vi "Get Settings.vi"(6 "wait for reply (T)":bool=TRUE, 8 "error in":errorcluster) -> (0 "error out":errorcluster, 1 "timed out?":bool, 3 "Main":T4={"Heat"={"KPтерм"=8.0, "TNтерм"=12.0, "KPниз"=4.0, "TNниз"=8.0, "COM ADC"="", "COM Termex"="", "KPдд"=4.0, "TNдд"=8.0, "Multiper"=1.0}, "Расчёты"={"Vm0"=8.0, "aa"=8.0, "bb"=8.0, "K0"=8.0, "A"=8.0, "B"=8.0}, "Видеосистема"=FALSE, "Anton Paar"={"IP adress"="192.168.0.110"}, "MIDA COM"="COM11"} {"Расчёты"."B" min=0.0 max=150.0 format="%.8f"; "Расчёты"."A" min=0.0 max=150.0 format="%.8f"; "Расчёты"."K0" min=0.0 max=150.0 format="%.2f"; "Расчёты"."bb" min=0.0 max=150.0 format="%.8f"; "Расчёты"."aa" min=0.0 max=150.0 format="%.8f"; "Расчёты"."Vm0" min=0.0 max=150.0 format="%.2f"; "Heat"."Multiper" min=0.0 max=150.0 format="%.2f"; "Heat"."TNдд" min=0.0 max=150.0 format="%.2f"; "Heat"."KPдд" min=0.0 max=150.0 format="%.2f"; "Heat"."TNниз" min=0.0 max=150.0 format="%.2f"; "Heat"."KPниз" min=0.0 max=150.0 format="%.2f"; "Heat"."TNтерм" min=0.0 max=150.0 format="%.2f"; "Heat"."KPтерм" min=0.0 max=150.0 format="%.2f"})   [LabVIEW 2023, in "Settings Master.lvlib"]
doc: "_____\nCreated using DQMH Event Scripter 6.1.0.128."
uses:
  Settings Master.lvlib
  Heat UI/Settings Type.ctl
  Drive/Calc_Type.ctl
  Menu/Setts.ctl
  Get Settings Argument--cluster.ctl
  Get Settings (Reply Payload)--cluster.ctl
  Heat UI/Heat UI.lvlib
  Drive/Drive.lvlib
  Menu/Menu.lvlib
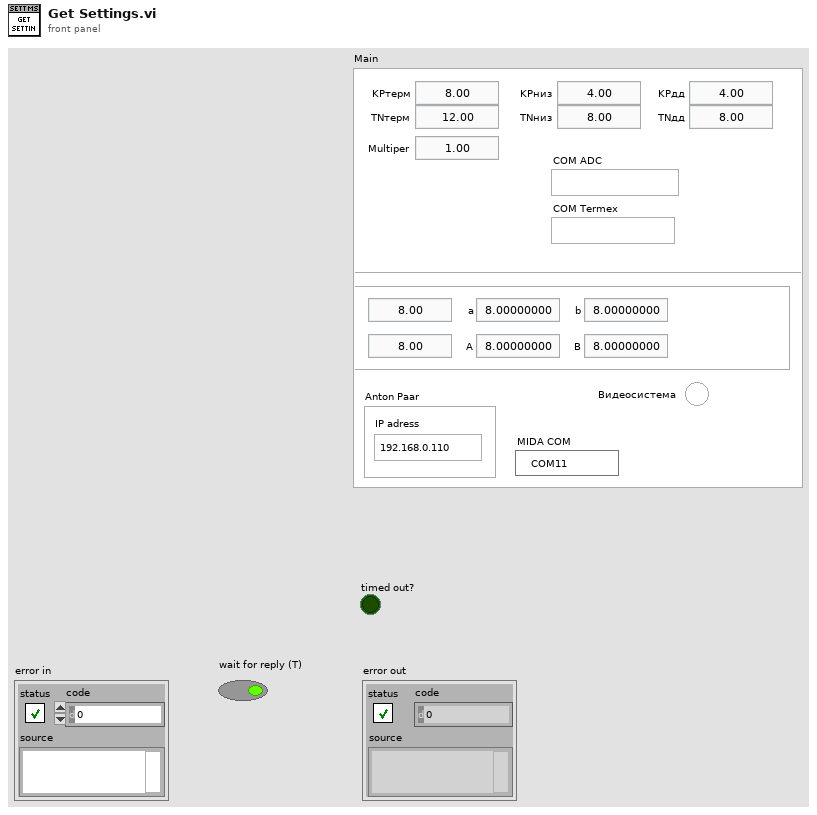
[diagram p1: front panel]
types:
  T1 = typedef "Heat UI.lvlib/Settings Type.ctl" = cluster{"KPтерм":dbl, "TNтерм":dbl, "KPниз":dbl, "TNниз":dbl, "COM ADC":refnum<visa-resource-name>, "COM Termex":refnum<visa-resource-name>, "KPдд":dbl, "TNдд":dbl, "Multiper":dbl}
  T2 = typedef "Drive.lvlib/Calc_Type.ctl" = cluster{"Vm0":dbl, "aa":dbl, "bb":dbl, "K0":dbl, "A":dbl, "B":dbl}
  T3 = typedef "Menu.lvlib/Setts.ctl" = cluster{"IP adress":string}
  T4 = cluster{"Heat":T1, "Расчёты":T2, "Видеосистема":bool, "Anton Paar":T3, "MIDA COM":refnum<visa-resource-name>}
  T5 = typedef "Settings Master.lvlib/Get Settings Argument--cluster.ctl" = cluster{"Wait Notifier":refnum<notifier>, "wait for reply":bool}
  T6 = typedef "Settings Master.lvlib/Request Events--cluster.ctl" = cluster{"Stop Module":refnum<user-event>, "Show Panel":refnum<user-event>, "Hide Panel":refnum<user-event>, "Get Module Execution Status":refnum<user-event>, "Show Diagram":refnum<user-event>, "Get Settings":refnum<user-event>, "SubPanel":refnum<user-event>}
  T7 = typedef "Settings Master.lvlib/Get Settings (Reply Payload)--cluster.ctl" = cluster{"Main":cluster{"Heat":T1, "Расчёты":T2, "Видеосистема":bool, "Anton Paar":T3, "MIDA COM":refnum<visa-resource-name>}, "error":errorcluster}
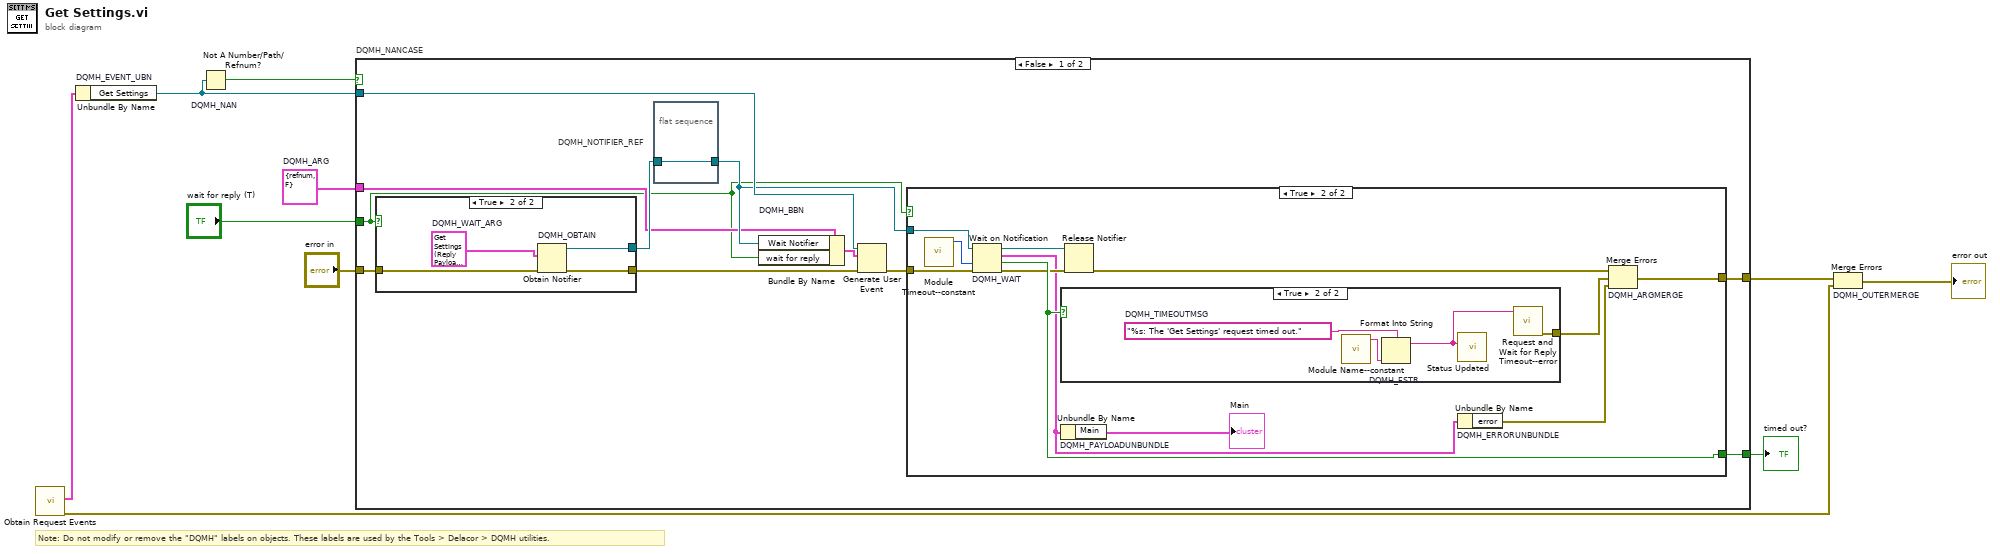
[diagram p0: block diagram]
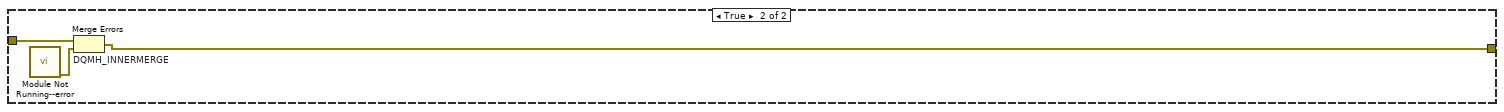
[diagram p5: hidden frame]
diagram:
  w4 = T5 {"Wait Notifier"=refnum, "wait for reply"=FALSE}  # DQMH_ARG
  # "Note: Do not modify or remove the \"DQMH\" labels on objects. These labels are used by the Tools > Delacor > DQMH utilities."
  n1 = call "Obtain Request Events.vi"() -> ("error out"=w2:errorcluster, "Settings Master Request Events"=w1:T6)  [unwired: 10 in]
  n2 = Unbundle By Name "DQMH_EVENT_UBN"(w1) -> ("Get Settings"=w8:refnum<user-event>)
  n3 = Not A Number/Path/Refnum? "DQMH_NAN"(number/path/refnum=w8) -> (NaN/Path/Refnum?=w7:bool)
  n4 = case "DQMH_NANCASE" shown="False" w7 {
    tunnel: "error in" -> [w21 w47]
    tunnel: w8 -> [w19 _]
    tunnel: [w16 w46] -> w5
    tunnel: [w17 _] -> w6
    tunnel: w4 -> [w12 _]
    tunnel: "wait for reply (T)" -> [w11 _]
    frame False {
      n5 = case shown="True" w11 {
        tunnel: w21 -> [w40 w44]
        tunnel: [w40 w43] -> w18
        tunnel: [_ w41] -> w14
        frame False {
        }
        frame True {
          w42 = T7 {"Main"={"Heat"={"KPтерм"=8.0, "TNтерм"=12.0, "KPниз"=4.0, "TNниз"=8.0, "COM ADC"="", "COM Termex"="", "KPдд"=4.0, "TNдд"=8.0, "Multiper"=1.0}, "Расчёты"={"Vm0"=8.0, "aa"=8.0, "bb"=8.0, "K0"=8.0, "A"=8.0, "B"=8.0}, "Видеосистема"=FALSE, "Anton Paar"={"IP adress"="192.168.0.110"}, "MIDA COM"="COM11"}, "error"={"status"=FALSE, "code"=0, "source"=""}}  # DQMH_WAIT_ARG
          n6 = Obtain Notifier "DQMH_OBTAIN"(notification data type=w42, error in (no error)=w44) -> (notifier out=w41:refnum<notifier>, error out=w43:errorcluster)  [unwired: 2 in, 1 out]
        }
      }
      n7 = flat-sequence "DQMH_NOTIFIER_REF" {
        tunnel: w14 -> [w22]
        tunnel: [w22] -> w13
        frame #0 {
        }
      }
      n8 = Bundle By Name "DQMH_BBN"(cluster=w12, "Wait Notifier"=w13, "wait for reply"=w11) -> (w15:T5)
      n9 = Generate User Event(user event=w19, event data cluster=w15, error in=w18) -> (error out=w20:errorcluster)  [unwired: 1 in, 1 out]
      n10 = case shown="True" w11 {
        tunnel: w20 -> [w23 w35]
        tunnel: w13 -> [_ w34]
        tunnel: [_ w32] -> w17
        tunnel: [w23 w31] -> w16
        frame False {
        }
        frame True {
          n11 = call "Module Timeout--constant.vi"() -> ("Module Timeout"=w25:i32)  [unwired: 11 in]
          n12 = Wait on Notification "DQMH_WAIT"(notifier=w34, timeout in ms (-1)=w25, error in (no error)=w35) -> (notifier out=w33:refnum<notifier>, notification=w26:T7, timed out?=w32:bool, error out=w30:errorcluster)  [unwired: 1 in]
          n13 = case shown="True" w32 {
            tunnel: [_ w37] -> w27
            frame False {
            }
            frame True {
              w39 = "%s: The 'Get Settings' request timed out."  # DQMH_TIMEOUTMSG
              n14 = call "Module Name--constant.vi"() -> ("Module Name"=w36:string)  [unwired: 11 in]
              n15 = Format Into String "DQMH_FSTR"(format string=w39, w36) -> (resulting string=w38:string)  [unwired: 2 in, 1 out]
              n16 = call "Status Updated.vi"("Status"=w38) -> ()  [unwired: 10 in, 1 out]
              n17 = call "Request and Wait for Reply Timeout--error.vi"("Error Message"=w38) -> ("error out"=w37:errorcluster)  [unwired: 10 in]
            }
          }
          n18 = Unbundle By Name "DQMH_PAYLOADUNBUNDLE"(w26) -> ("Main"=→"Main":T4)
          n19 = Release Notifier(notifier=w33, error in (no error)=w30) -> (error out=w29:errorcluster)  [unwired: 1 in, 2 out]
          n20 = Unbundle By Name "DQMH_ERRORUNBUNDLE"(w26) -> ("error"=w28:errorcluster)
          n21 = Merge Errors "DQMH_ARGMERGE"(w29, w27, w28) -> (w31:errorcluster)
        }
      }
    }
    frame True {
      n22 = call "Module Not Running--error.vi"() -> ("error out"=w45:errorcluster)  [unwired: 11 in]
      n23 = Merge Errors "DQMH_INNERMERGE"(w47, w45) -> (w46:errorcluster)
    }
  }
  "timed out?" <- w6
  n24 = Merge Errors "DQMH_OUTERMERGE"(w5, w2) -> (→"error out":errorcluster)
